vi "notions_cles.vi"(0 "dettes":dbl, 1 "Argent ventes":dbl, 2 "CA":dbl, 3 "Impots":dbl, 4 "Calculs button":bool) -> (5 "notions_cles":dbl[](array[numeric]))   [LabVIEW 2024]
uses:
  <vilib>/express/express shared/transition.llb/Dynamic To Waveform Array.vi
  <vilib>/express/express signal manip/GetorSetDDTAttributes/Set DDT Attributes/SetT0.vi
  <vilib>/express/express shared/transition.llb/Waveform Array To Dynamic.vi
  <vilib>/express/express signal manip/GetorSetDDTAttributes/Set DDT Attributes/Set DDT Properties.xnode
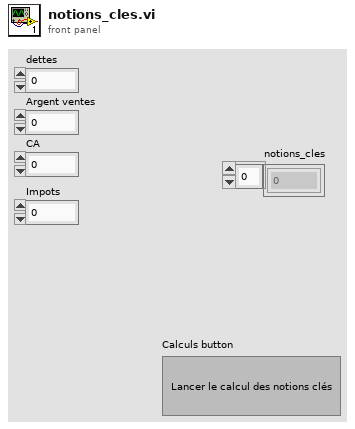
[diagram p1: front panel]
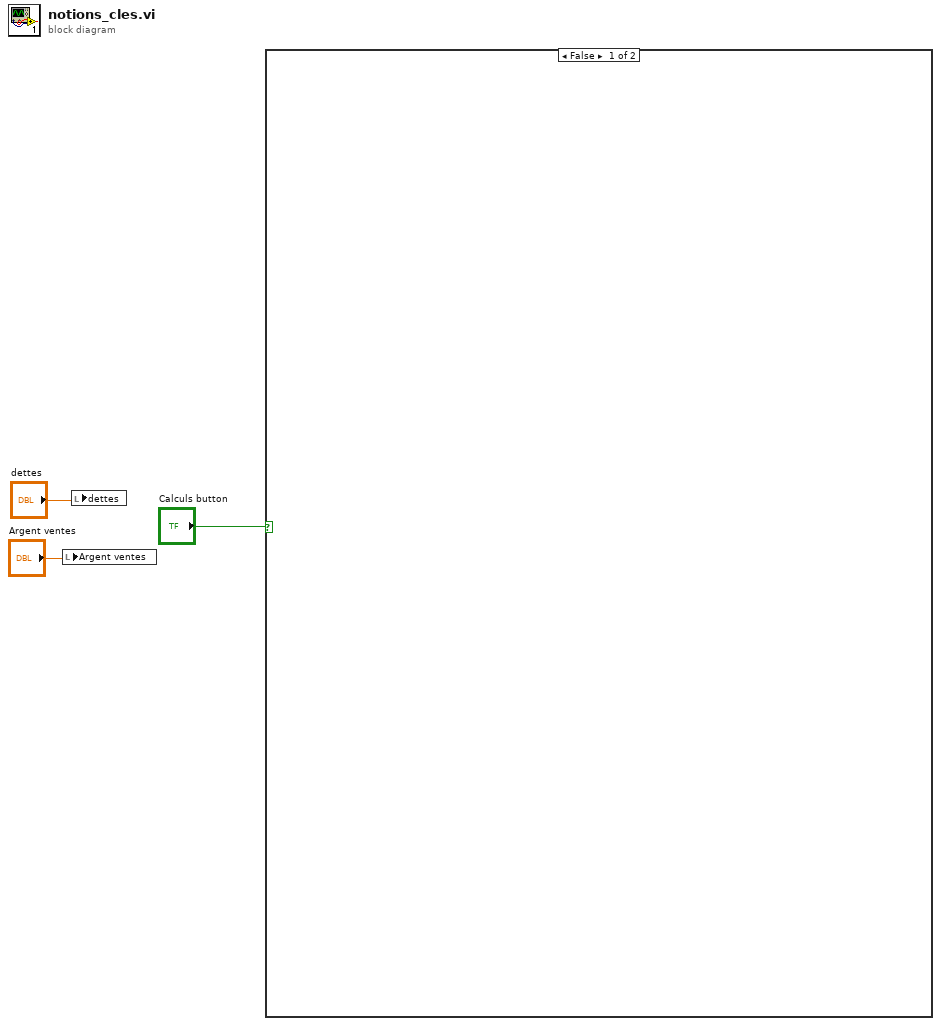
[diagram p0: block diagram]
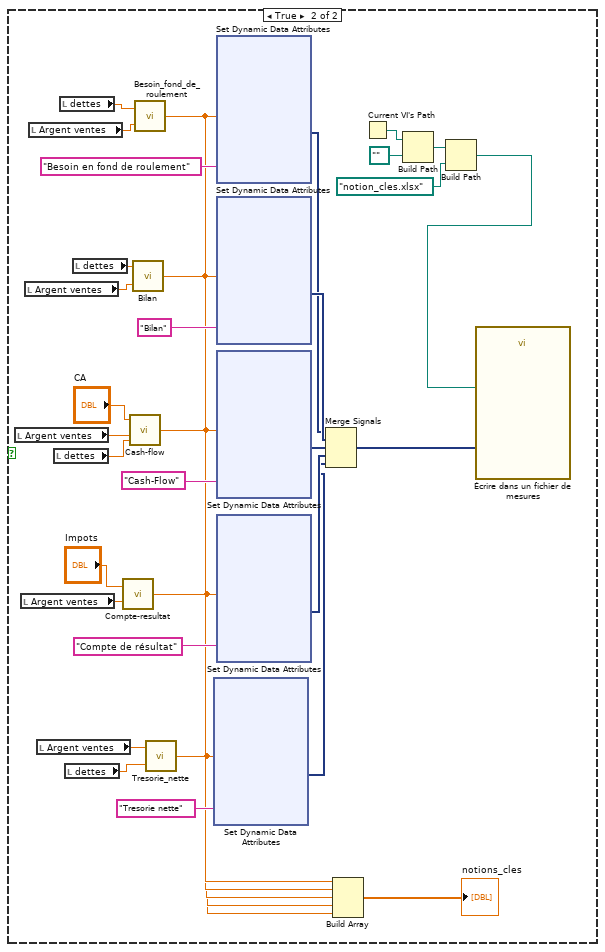
[diagram p2: hidden frame]
diagram:
  n1 = local write "Argent ventes"("Argent ventes") -> ()
  n2 = local write "dettes"("dettes") -> ()
  n3 = case shown="False" "Calculs button" {
    frame False {
    }
    frame True {
      n4 = local read "Argent ventes"() -> (w21:dbl)
      n5 = local read "Argent ventes"() -> (w18:dbl)
      n6 = local read "Argent ventes"() -> (w23:dbl)
      n7 = local read "Argent ventes"() -> (w25:dbl)
      n8 = local read "Argent ventes"() -> (w17:dbl)
      n9 = local read "dettes"() -> (w20:dbl)
      n10 = local read "dettes"() -> (w26:dbl)
      n11 = local read "dettes"() -> (w16:dbl)
      n12 = local read "dettes"() -> (w24:dbl)
      n13 = call "Compte-resultat.vi"("Argent ventes"=w18, "Impots"="Impots") -> ("Compte résultat"=w10:dbl)
      n14 = call "Cash-flow.vi"("Dettes"=w20, "Argent ventes"=w21, "CA"="CA") -> ("Cash Flow"=w11:dbl)
      n15 = call "Bilan.vi"("Argent ventes"=w23, "Dettes"=w24) -> ("Bilan"=w12:dbl)
      n16 = call "Besoin_fond_de_roulement.vi"("Argent ventes"=w25, "dettes"=w26) -> ("BFR"=w13:dbl)
      n17 = call "Tresorie_nette.vi"("Dettes"=w16, "Argent ventes"=w17) -> ("tresorire nette"=w9:dbl)
      n18 = xnode "Set Dynamic Data Attributes"("Signals In"=w9, "Signal Name"="Tresorie nette") -> ("Signals Out"=w33:dynamicdata)  [unwired: 2 in, 1 out]
      n19 = xnode "Set Dynamic Data Attributes"("Signals In"=w13, "Signal Name"="Besoin en fond de roulement") -> ("Signals Out"=w32:dynamicdata)  [unwired: 2 in, 1 out]
      n20 = xnode "Set Dynamic Data Attributes"("Signals In"=w12, "Signal Name"="Bilan") -> ("Signals Out"=w36:dynamicdata)  [unwired: 2 in, 1 out]
      n21 = xnode "Set Dynamic Data Attributes"("Signals In"=w11, "Signal Name"="Cash-Flow") -> ("Signals Out"=w35:dynamicdata)  [unwired: 2 in, 1 out]
      n22 = xnode "Set Dynamic Data Attributes"("Signals In"=w10, "Signal Name"="Compte de résultat") -> ("Signals Out"=w34:dynamicdata)  [unwired: 2 in, 1 out]
      n23 = Merge Signals(w32, w36, w35, w34, w33) -> (w15:dynamicdata)
      n24 = Build Array(w13, w12, w11, w10, w9) -> (→"notions_cles":dbl[])
      n25 = Current VI's Path() -> (path=w8:path)
      n26 = Build Path(base path=w8, name or relative path=path "..") -> (appended path=w5:path)
      n27 = Build Path(base path=w5, name or relative path=path "notion_cles.xlsx" ("Filename")) -> (appended path=w4:path)
      n28 = call "Écrire dans un fichier de mesures"("Signals"=w15, "Filename"=w4) -> ()  [unwired: 15 in, 3 out]
    }
  }
